vi "Build Data Frame.vi"(4 "Payload Class (Data)":T2=enum."Data", 5 "Destination (None)":T1, 6 "Payload ID (0)":u16, 8 "error in (no error)":errorcluster, 10 "Options (0)":u32, 11 "Payload (Empty String)":string) -> (0 "error out":errorcluster, 3 "Frame":variant)   [LabVIEW 2023]
doc: "This VI takes in payload and metadata as controls and generates a properly formed data frame out of it. The output is a variant and must be converted to traditional data before it is unpacked.\n\nThis VI exhibits standard error in and error out functionality and returns an empty variant in case of error."
uses:
  Type Definitions/Payload Class.ctl
  Type Definitions/Device.ctl
  Type Definitions/Data Frame.ctl
  Type Definitions/Data Frame Header.ctl
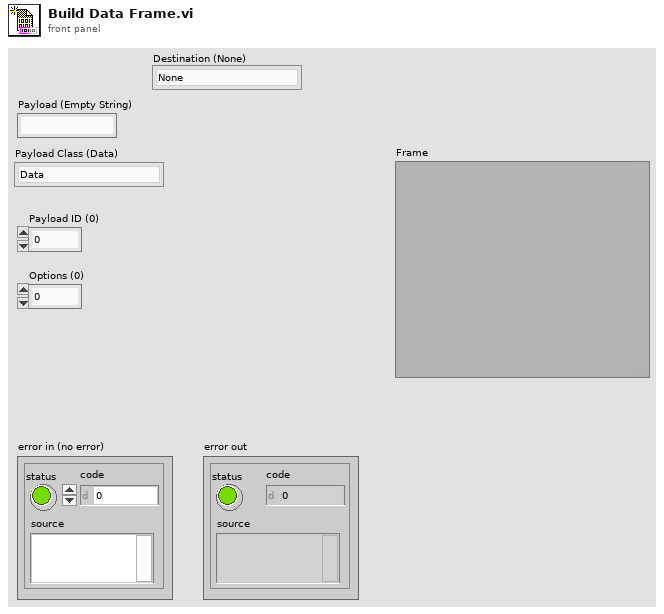
[diagram p1: front panel]
types:
  T1 = typedef "Device.ctl" = enum32{"None", "Exec", "Aux1", "Aux2", "Aux3"}
  T2 = typedef "Payload Class.ctl" = enum16{"System State", "Parameters", "Metadata", "Software Monitor", "Data", "Commands"}
  T3 = typedef "Data Frame.ctl" = cluster{"Frame Header":T4, "Payload":string, "CRC":u32}
  T4 = typedef "Data Frame Header.ctl" = cluster{"Sync":u32, "Time":dbl, "Nanosecond Counter":i64, "Payload Class":T2, "Payload ID":u16, "Counter":i32, "Options":u32, "Source":T1, "Destination":T1}
  T5 = typedef "LVDateTimeRec.ctl" = cluster{"fractional second":dbl, "second":i32, "minute":i32, "hour":i32, "day of month":i32, "month":i32, "year":i32, "day of week":i32, "day of year":i32, "DST":i32}
  T6 = cluster{"Sync":u32, dbl, i64, "Payload Class (Data)":T2, "Payload ID (0)":u16, "Count":i32, "Options (0)":u32, "Device":T1, "Destination (None)":T1, "Payload (Empty String)":string}
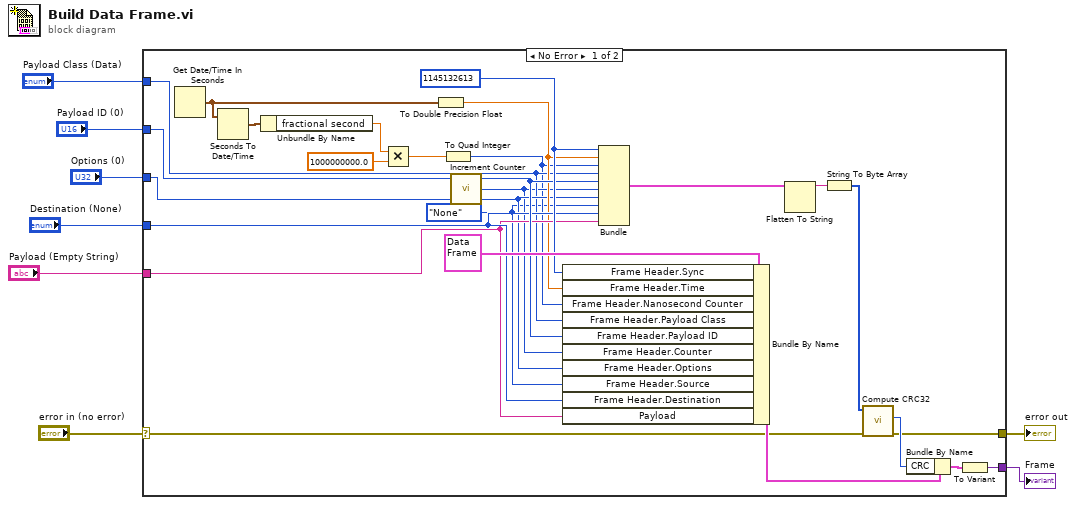
[diagram p0: block diagram]
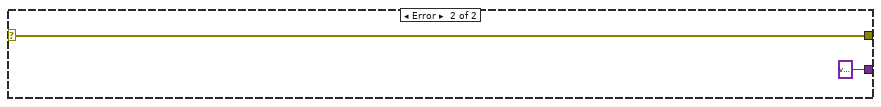
[diagram p2: hidden frame]
diagram:
  n1 = case shown="No Error" "error in (no error)" {
    selector: "error in (no error)" -> [w10 w35]
    tunnel: "Payload Class (Data)" -> [w19 _]
    tunnel: "Payload ID (0)" -> [w31 _]
    tunnel: "Options (0)" -> [w21 _]
    tunnel: "Destination (None)" -> [w30 _]
    tunnel: "Payload (Empty String)" -> [w25 _]
    tunnel: [w18 variant ("Variant")] -> w6
    tunnel: [w20 w35] -> w7
    frame No Error {
      w9 = Device."None" ("Device")
      w32 = u32 1145132613 ("Sync")
      n2 = Get Date/Time In Seconds() -> (seconds since 1Jan1904=w16:timestamp)
      n3 = Seconds To Date/Time(time stamp (now)=w16) -> (date time rec=w15:T5)  [unwired: 1 in]
      n4 = Unbundle By Name(w15) -> ("fractional second"=w14:dbl)
      n5 = Multiply(x=w14, y=1000000000.0) -> (x*y=w12:dbl)
      n6 = To Double Precision Float(number=w16) -> (double precision float=w22:dbl)
      n7 = To Quad Integer(1:w12) -> (0:w11:i64)
      n8 = call "Increment Counter.vi"() -> ("Count"=w17:i32)  [unwired: 5 in]
      n9 = Bundle By Name(cluster=T3 {"Frame Header"={"Sync"=0, "Time"=0.0, "Nanosecond Counter"=0, "Payload Class"=enum."System State", "Payload ID"=0, "Counter"=0, "Options"=0, "Source"=enum."None", "Destination"=enum."None"}, "Payload"="", "CRC"=0} ("Frame"), "Frame Header.Sync"=w32, "Frame Header.Time"=w22, "Frame Header.Nanosecond Counter"=w11, "Frame Header.Payload Class"=w19, "Frame Header.Payload ID"=w31, "Frame Header.Counter"=w17, "Frame Header.Options"=w21, "Frame Header.Source"=w9, "Frame Header.Destination"=w30, "Payload"=w25) -> (w24:T3)
      n10 = Bundle("Sync"=w32, w22, w11, "Payload Class (Data)"=w19, "Payload ID (0)"=w31, "Count"=w17, "Options (0)"=w21, "Device"=w9, "Destination (None)"=w30, "Payload (Empty String)"=w25) -> (w23:T6)  [unwired: 1 in]
      n11 = Flatten To String(anything=w23) -> (data string=w26:string)  [unwired: 3 in, 2 out]
      n12 = String To Byte Array(string=w26) -> (unsigned byte array=w29:u8[])
      n13 = call "Compute CRC32.vi"("error in (no error)"=w10, "inputArray"=w29) -> ("error out"=w20:errorcluster, "CRC32Value"=w28:u32)  [unwired: 8 in]
      n14 = Bundle By Name(cluster=w24, "CRC"=w28) -> (w27:T3)
      n15 = To Variant(anything=w27) -> (Variant=w18:variant)
    }
    frame Error {
    }
  }
  "Frame" <- w6
  "error out" <- w7
